vi "spybotauto.vi"   [LabVIEW 2015]
uses:
  <vilib>/Rock Robotics/WPI/CAN/TalonSRX/WPI_CANTalonSRX_APIControlMode.ctl
types:
  T1 = typedef "WPI_MotorControlDeviceRef.ctl" = cluster{"DeviceStatus":errorcluster, "Type":T2, "PWM":cluster{"PWM Channel":T3, "DeadBand":T4}, "CAN":cluster{"Device Number":u8, "Control Mode":T5, "Semaphore":T6, "Max Vout":dbl, "TalonSRX Control Mode":T7}, "Invert":bool}
  T2 = typedef "WPI_MotorControlType.ctl" = enum16{"PWM", "CAN", "CANTalonSRX"}
  T3 = typedef "FPGA_DIOPWMChannel.ctl" = enum8{"PWM 0", "PWM 1", "PWM 2", "PWM 3", "PWM 4", "PWM 5", "PWM 6", "PWM 7", "PWM 8", "PWM 9", "PWM MXP 0", "PWM MXP 1", "PWM MXP 2", "PWM MXP 3", "PWM MXP 4", "PWM MXP 5", "PWM MXP 6", "PWM MXP 7", "PWM MXP 8", "PWM MXP 9", "Invalid"}
  T4 = typedef "WPI_PWMDeadband.ctl" = cluster{"Name":string, "maxPositivePwm":i32, "minPositivePwm":i32, "centerPwm":i32, "maxNegativePwm":i32, "minNegativePwm":i32, "angularRange":u16}
  T5 = typedef "WPI_CANJaguar_ControlMode.ctl" = enum8{"Percent VBus", "Current", "Speed", "Position", "Voltage"}
  T6 = typedef "Semaphore RefNum" = refnum<k1>
  T7 = typedef "WPI_CANTalonSRX_APIControlMode.ctl" = enum8{"Percent VBus", "Speed", "Position", "Slave", "Unchanged / Invalid", "Voltage Compensation", "Current", "Motion Profile"}
  T8 = typedef "WPI_EncoderDevRef.ctl" = cluster{"DevStatus":errorcluster, "EncoderIndex":T9, "CounterIndex":T10, "DistancePerCount":dbl, "Decoding Type":T11}
  T9 = typedef "FPGA_EncoderIdx.ctl" = enum8{"Enc 0", "Enc 1", "Enc 2", "Enc 3", "Enc 4", "Enc 5", "Enc 6", "Enc 7", "Invalid"}
  T10 = typedef "FPGA_CounterCtrSystemIndex.ctl" = enum8{"Ctr 0", "Ctr 1", "Ctr 2", "Ctr 3", "Ctr 4", "Ctr 5", "Ctr 6", "Ctr 7", "Invalid"}
  T11 = typedef "WPI_EncoderType.ctl" = enum16{"1x", "2x", "4x"}
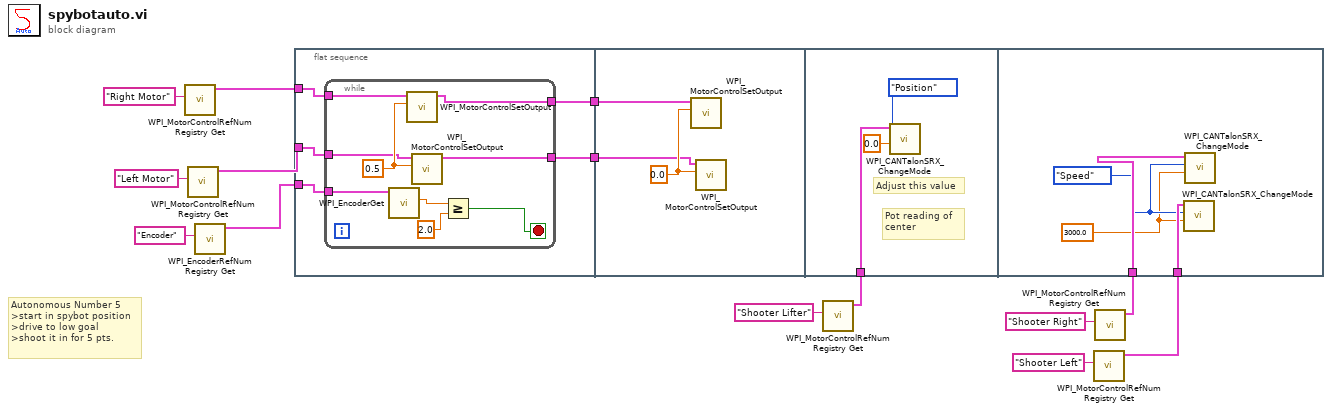
[diagram p0: block diagram]
diagram:
  # "Autonomous Number 5\n>start in spybot position\n>drive to low goal\n>shoot it in for 5 pts."
  n1 = call <vilib>:"WPI_MotorControlRefNum Registry Get.vi"("refnum name"="Right Motor") -> ("MotorControlDevRef"=w11:T1)  [unwired: 9 in, 1 out]
  n2 = call <vilib>:"WPI_MotorControlRefNum Registry Get.vi"("refnum name"="Left Motor") -> ("MotorControlDevRef"=w12:T1)  [unwired: 9 in, 1 out]
  n3 = call <vilib>:"WPI_EncoderRefNum Registry Get.vi"("refnum name"="Encoder") -> ("EncoderDevRef"=w9:T8)  [unwired: 9 in, 1 out]
  n4 = flat-sequence {
    tunnel: w12 -> [w19]
    tunnel: w11 -> [w18]
    tunnel: w9 -> [w17]
    tunnel: [w16] -> w2
    tunnel: [w15] -> w1
    tunnel: w2 -> [w30]
    tunnel: w1 -> [w29]
    tunnel: w7 -> [w34]
    tunnel: w4 -> [w38]
    tunnel: w3 -> [w37]
    frame #0 {
      n5 = while {
        tunnel: w19 -> [w27]
        tunnel: w18 -> [w26]
        tunnel: w17 -> [w25]
        tunnel: [w21] -> w16
        tunnel: [w20] -> w15
        stop <- w22 stop-if-true
        w28 = 0.5 ("Output")
        n6 = call <vilib>:"WPI_EncoderGet.vi"("EncoderDevRef"=w25) -> ("Distance"=w24:dbl)  [unwired: 5 in, 5 out]
        n7 = call <vilib>:"WPI_MotorControlSetOutput.vi"("Output"=w28, "MotorControlDevRef"=w26) -> ("MotorControlDevRef"=w20:T1)  [unwired: 7 in, 2 out]
        n8 = call <vilib>:"WPI_MotorControlSetOutput.vi"("Output"=w28, "MotorControlDevRef"=w27) -> ("MotorControlDevRef"=w21:T1)  [unwired: 7 in, 2 out]
        n9 = Greater Or Equal?(x=w24, y=2.0) -> (x >= y?=w22:bool)
      }
    }
    frame #1 {
      w31 = 0.0 ("Output")
      n10 = call <vilib>:"WPI_MotorControlSetOutput.vi"("Output"=w31, "MotorControlDevRef"=w29) -> ()  [unwired: 7 in, 3 out]
      n11 = call <vilib>:"WPI_MotorControlSetOutput.vi"("Output"=w31, "MotorControlDevRef"=w30) -> ()  [unwired: 7 in, 3 out]
    }
    frame #2 {
      # "Pot reading of \ncenter"
      # "Adjust this value"
      n12 = call <vilib>:"WPI_CANTalonSRX_ChangeMode.vi"("Output"=0.0, "Control Mode"=WPI_CANTalonSRX_APIControlMode."Position", "CAN Talon SRX Ref"=w34) -> ()  [unwired: 7 in, 2 out]
    }
    frame #3 {
      w35 = 3000.0
      w36 = WPI_CANTalonSRX_APIControlMode."Speed" ("Control Mode")
      n13 = call <vilib>:"WPI_CANTalonSRX_ChangeMode.vi"("Output"=w35, "Control Mode"=w36, "CAN Talon SRX Ref"=w37) -> ()  [unwired: 7 in, 2 out]
      n14 = call <vilib>:"WPI_CANTalonSRX_ChangeMode.vi"("Output"=w35, "Control Mode"=w36, "CAN Talon SRX Ref"=w38) -> ()  [unwired: 7 in, 2 out]
    }
  }
  n15 = call <vilib>:"WPI_MotorControlRefNum Registry Get.vi"("refnum name"="Shooter Lifter") -> ("MotorControlDevRef"=w7:T1)  [unwired: 9 in, 1 out]
  n16 = call <vilib>:"WPI_MotorControlRefNum Registry Get.vi"("refnum name"="Shooter Left") -> ("MotorControlDevRef"=w3:T1)  [unwired: 9 in, 1 out]
  n17 = call <vilib>:"WPI_MotorControlRefNum Registry Get.vi"("refnum name"="Shooter Right") -> ("MotorControlDevRef"=w4:T1)  [unwired: 9 in, 1 out]
